vi "TCP-Parse Key.vi"(8 "error in (no error)":errorcluster, 10 "Value":string, 11 "Key":string) -> (0 "error out":errorcluster)   [LabVIEW 2015]
uses:
  DAQ Engine VIs/PXI Globals.vi
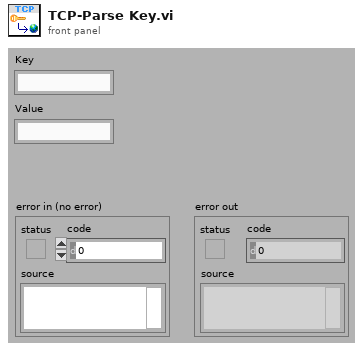
[diagram p1: front panel]
types:
  T1 = typedef "Counter Params.ctl" = cluster{"Counter":tag, "Hi ticks":u32, "Low ticks":u32, "Idle state":i32, "Delay ticks":u32}
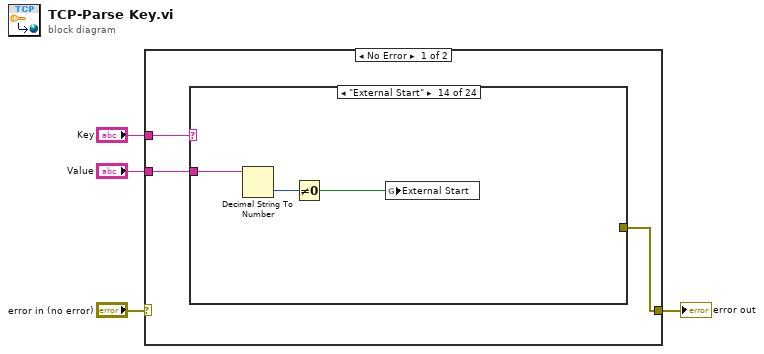
[diagram p0: block diagram]
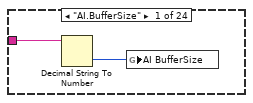
[diagram p2: hidden frame]
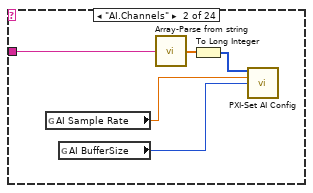
[diagram p3: hidden frame]
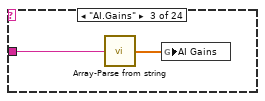
[diagram p4: hidden frame]
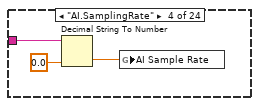
[diagram p5: hidden frame]
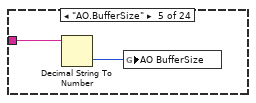
[diagram p6: hidden frame]
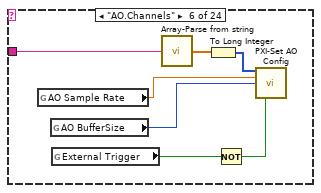
[diagram p7: hidden frame]
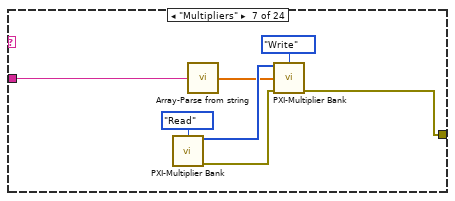
[diagram p8: hidden frame]
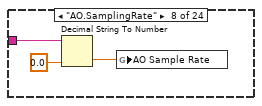
[diagram p9: hidden frame]
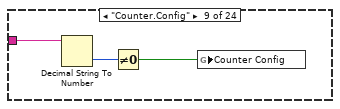
[diagram p10: hidden frame]
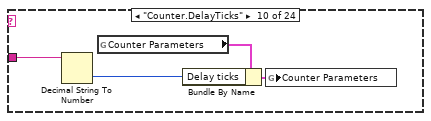
[diagram p11: hidden frame]
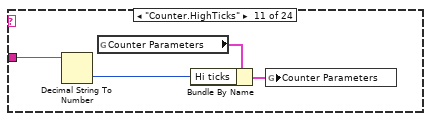
[diagram p12: hidden frame]
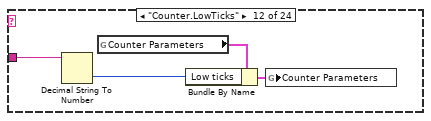
[diagram p13: hidden frame]
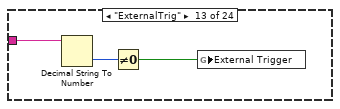
[diagram p14: hidden frame]
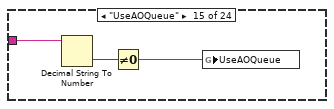
[diagram p15: hidden frame]
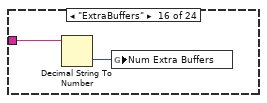
[diagram p16: hidden frame]
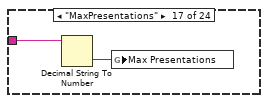
[diagram p17: hidden frame]
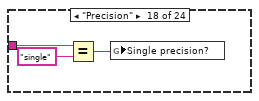
[diagram p18: hidden frame]
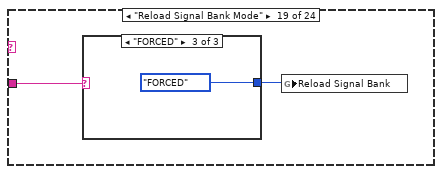
[diagram p19: hidden frame]
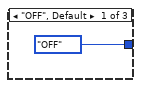
[diagram p20: hidden frame]
diagram:
  n1 = case shown="No Error" "error in (no error)" {
    selector: "error in (no error)" -> [_ w91]
    tunnel: "Key" -> [w7 _]
    tunnel: "Value" -> [w6 _]
    tunnel: [w5 w91] -> w1
    frame No Error {
      n2 = case shown="\"External Start\"" w7 {
        selector: w7 -> [_ _ _ _ _ _ _ _ _ _ _ _ _ _ _ _ _ _ _ _ _ _ _ w88]
        tunnel: w6 -> [w9 w12 w16 w19 w21 w26 w30 w38 w41 w45 w49 w53 w56 w59 w62 w64 w66 w69 w71 w77 w79 w82 w85 _]
        tunnel: [_ _ _ _ _ _ w31 _ _ _ _ _ _ _ _ _ _ _ _ _ _ _ _ w86] -> w5
        frame "AI.BufferSize" {
          n3 = Decimal String To Number(string=w9) -> (number=w8:i32)  [unwired: 2 in, 1 out]
          n4 = global write "PXI Globals.vi" "AI BufferSize"(w8) -> ()
        }
        frame "AI.Channels" {
          n5 = global read "PXI Globals.vi" "AI Sample Rate"() -> (w14:dbl)
          n6 = global read "PXI Globals.vi" "AI BufferSize"() -> (w13:i32)
          n7 = call "Array-Parse from string.vi"("String"=w12) -> ("Array"=w11:dbl[])  [unwired: 13 in, 1 out]
          n8 = To Long Integer(number=w11) -> (32bit integer=w10:i32[])
          n9 = call "PXI-Set AI Config.vi"("AI Channels"=w10, "Sampling Rate (Hz)"=w14, "Buffer Size"=w13) -> ()  [unwired: 12 in, 1 out]
        }
        frame "AI.Gains" {
          n10 = call "Array-Parse from string.vi"("String"=w16) -> ("Array"=w15:dbl[])  [unwired: 13 in, 1 out]
          n11 = global write "PXI Globals.vi" "AI Gains"(w15) -> ()
        }
        frame "AI.SamplingRate" {
          n12 = Decimal String To Number(string=w19, default (0L)=0.0) -> (number=w17:dbl)  [unwired: 1 in, 1 out]
          n13 = global write "PXI Globals.vi" "AI Sample Rate"(w17) -> ()
        }
        frame "AO.BufferSize" {
          n14 = Decimal String To Number(string=w21) -> (number=w20:i32)  [unwired: 2 in, 1 out]
          n15 = global write "PXI Globals.vi" "AO BufferSize"(w20) -> ()
        }
        frame "AO.Channels" {
          n16 = global read "PXI Globals.vi" "AO Sample Rate"() -> (w28:dbl)
          n17 = global read "PXI Globals.vi" "AO BufferSize"() -> (w27:i32)
          n18 = global read "PXI Globals.vi" "External Trigger"() -> (w23:bool)
          n19 = call "Array-Parse from string.vi"("String"=w26) -> ("Array"=w25:dbl[])  [unwired: 13 in, 1 out]
          n20 = To Long Integer(number=w25) -> (32bit integer=w24:i32[])
          n21 = Not(x=w23) -> (.not. x?=w22:bool)
          n22 = call "PXI-Set AO Config.vi"("AO Channels"=w24, "Sampling Rate (Hz)"=w28, "Buffer Size"=w27, "Regenerate"=w22) -> ()  [unwired: 11 in, 1 out]
        }
        frame "Multipliers" {
          n23 = call "PXI-Multiplier Bank.vi"("Action"=enum16{"Init", "Write", "Read"}."Read") -> ("Channels"=w33:i32[], "error out"=w32:errorcluster)  [unwired: 12 in, 1 out]
          n24 = call "Array-Parse from string.vi"("String"=w30) -> ("Array"=w29:dbl[])  [unwired: 13 in, 1 out]
          n25 = call "PXI-Multiplier Bank.vi"("AO Channels"=w33, "Action"=enum16{"Init", "Write", "Read"}."Write", "Multipliers"=w29, "error in (no error)"=w32) -> ("error out"=w31:errorcluster)  [unwired: 9 in, 2 out]
        }
        frame "AO.SamplingRate" {
          n26 = Decimal String To Number(string=w38, default (0L)=0.0) -> (number=w36:dbl)  [unwired: 1 in, 1 out]
          n27 = global write "PXI Globals.vi" "AO Sample Rate"(w36) -> ()
        }
        frame "Counter.Config" {
          n28 = Decimal String To Number(string=w41) -> (number=w40:i32)  [unwired: 2 in, 1 out]
          n29 = Not Equal To 0?(x=w40) -> (x != 0?=w39:bool)
          n30 = global write "PXI Globals.vi" "Counter Config"(w39) -> ()
        }
        frame "Counter.DelayTicks" {
          n31 = Decimal String To Number(string=w45) -> (number=w43:i32)  [unwired: 2 in, 1 out]
          n32 = global read "PXI Globals.vi" "Counter Parameters"() -> (w44:T1)
          n33 = Bundle By Name(cluster=w44, "Delay ticks"=w43) -> (w42:T1)
          n34 = global write "PXI Globals.vi" "Counter Parameters"(w42) -> ()
        }
        frame "Counter.HighTicks" {
          n35 = Decimal String To Number(string=w49) -> (number=w47:i32)  [unwired: 2 in, 1 out]
          n36 = global read "PXI Globals.vi" "Counter Parameters"() -> (w48:T1)
          n37 = Bundle By Name(cluster=w48, "Hi ticks"=w47) -> (w46:T1)
          n38 = global write "PXI Globals.vi" "Counter Parameters"(w46) -> ()
        }
        frame "Counter.LowTicks" {
          n39 = Decimal String To Number(string=w53) -> (number=w51:i32)  [unwired: 2 in, 1 out]
          n40 = global read "PXI Globals.vi" "Counter Parameters"() -> (w52:T1)
          n41 = Bundle By Name(cluster=w52, "Low ticks"=w51) -> (w50:T1)
          n42 = global write "PXI Globals.vi" "Counter Parameters"(w50) -> ()
        }
        frame "ExternalTrig" {
          n43 = Decimal String To Number(string=w56) -> (number=w55:i32)  [unwired: 2 in, 1 out]
          n44 = Not Equal To 0?(x=w55) -> (x != 0?=w54:bool)
          n45 = global write "PXI Globals.vi" "External Trigger"(w54) -> ()
        }
        frame "External Start" {
          n46 = Decimal String To Number(string=w59) -> (number=w58:i32)  [unwired: 2 in, 1 out]
          n47 = Not Equal To 0?(x=w58) -> (x != 0?=w57:bool)
          n48 = global write "PXI Globals.vi" "External Start"(w57) -> ()
        }
        frame "UseAOQueue" {
          n49 = Decimal String To Number(string=w62) -> (number=w61:i32)  [unwired: 2 in, 1 out]
          n50 = Not Equal To 0?(x=w61) -> (x != 0?=w60:bool)
          n51 = global write "PXI Globals.vi" "UseAOQueue"(w60) -> ()
        }
        frame "ExtraBuffers" {
          n52 = Decimal String To Number(string=w64) -> (number=w63:i32)  [unwired: 2 in, 1 out]
          n53 = global write "PXI Globals.vi" "Num Extra Buffers"(w63) -> ()
        }
        frame "MaxPresentations" {
          n54 = Decimal String To Number(string=w66) -> (number=w65:i32)  [unwired: 2 in, 1 out]
          n55 = global write "PXI Globals.vi" "Max Presentations"(w65) -> ()
        }
        frame "Precision" {
          n56 = Equal?(x=w69, y="single") -> (x = y?=w67:bool)
          n57 = global write "PXI Globals.vi" "Single precision?"(w67) -> ()
        }
        frame "Reload Signal Bank Mode" {
          n58 = case shown="\"FORCED\"" w71 {
            tunnel: [enum32{"OFF", "ENABLED", "FORCED"}."OFF" ("Reload Signal Bank") enum32{"OFF", "ENABLED", "FORCED"}."ENABLED" ("Reload Signal Bank") enum32{"OFF", "ENABLED", "FORCED"}."FORCED" ("Reload Signal Bank")] -> w70
            frame "OFF", Default {
            }
            frame "ENABLED" {
            }
            frame "FORCED" {
            }
          }
          n59 = global write "PXI Globals.vi" "Reload Signal Bank"(w70) -> ()
        }
        frame "SendData" {
          n60 = Decimal String To Number(string=w77) -> (number=w76:i32)  [unwired: 2 in, 1 out]
          n61 = Not Equal To 0?(x=w76) -> (x != 0?=w75:bool)
          n62 = global write "PXI Globals.vi" "Send Data"(w75) -> ()
        }
        frame "SkipSamples" {
          n63 = Decimal String To Number(string=w79) -> (number=w78:i32)  [unwired: 2 in, 1 out]
          n64 = global write "PXI Globals.vi" "Skip Samples"(w78) -> ()
        }
        frame "Stop on MaxPresentations" {
          n65 = Decimal String To Number(string=w82) -> (number=w81:i32)  [unwired: 2 in, 1 out]
          n66 = Not Equal To 0?(x=w81) -> (x != 0?=w80:bool)
          n67 = global write "PXI Globals.vi" "Stop on MaxPresentations"(w80) -> ()
        }
        frame "TCPData" {
          n68 = Decimal String To Number(string=w85) -> (number=w84:i32)  [unwired: 2 in, 1 out]
          n69 = Not Equal To 0?(x=w84) -> (x != 0?=w83:bool)
          n70 = global write "PXI Globals.vi" "TCPData"(w83) -> ()
        }
        frame "ZZZ", Default {
          n71 = Format Into String(format string="Unexpected key: %s", w88) -> (resulting string=w87:string)  [unwired: 2 in, 1 out]
          n72 = call <vilib>:"Error Cluster From Error Code.vi"("error message (\"\")"=w87, "error code (0)"=-6000) -> ("error out"=w86:errorcluster)  [unwired: 7 in]
        }
      }
    }
    frame Error {
    }
  }
  "error out" <- w1
